vi "Null Value.vi"() -> (0 "Null":variant)   [LabVIEW 2019, in "JKI JSON Serialization.lvlib"]
doc: "JKI JSON 1.1.10.37\nTomi Maila - JKI\nCopyright (c) 2017, JKI"
uses:
  JKI JSON Serialization.lvlib
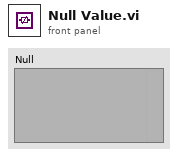
[diagram p1: front panel]
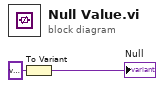
[diagram p0: block diagram]
diagram:
  n1 = To Variant(anything=variant ("variant")) -> (Variant=→"Null":variant)
